vi "Lookup Channel Info.vi"(8 "error in (no error)":errorcluster, 10 "Channel Name":string, 11 "VolatusAPI in":refnum<class "VolatusAPI.lvclass">) -> (0 "error out":errorcluster, 1 "Local":bool, 2 "Channel Info":T1, 3 "VolatusAPI out":refnum<class "VolatusAPI.lvclass">, 4 "Index":i32)   [LabVIEW 2020, in "Volatus.lvlib" / "VolatusAPI.lvclass"]
uses:
  VolatusAPI.lvclass
  lv-vecto/Vecto/Channel Info.ctl
  VolatusAPI.lvclass/VolatusAPI.ctl
  VolatusConfig/VolatusConfig.lvlib
  VolatusConfig/Meta Type.ctl
  lv-cdm/CDM-Config/Config Filter/Config Lookup.lvclass
  VolatusConfig/VolatusConfigElement/VolatusConfigElement.lvclass
  VolatusConfig/Group/Group Config.lvclass
  VolatusConfig/Node/Node Config.lvclass
  C:/dev/lv20CE/relink/lv-volatus/VolatusConfig/VolatusConfigElement/VolatusConfigElement.lvclass
  C:/dev/lv20CE/relink/lv-volatus/VolatusConfig/Node/Node Config.lvclass
  lv-vecto/VectoConfig/VectoConfig.lvlib
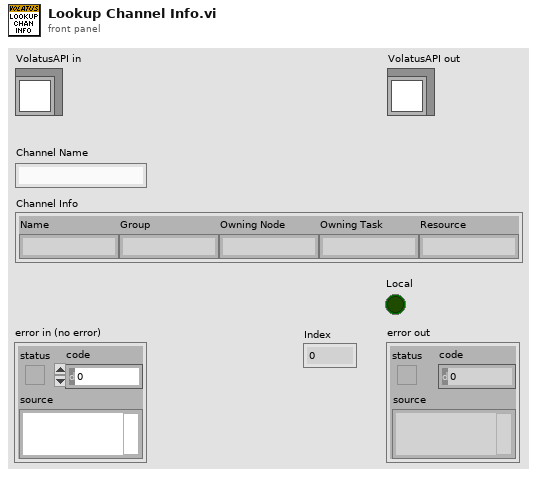
[diagram p1: front panel]
types:
  T1 = typedef "VectoConfig.lvlib/Channel Info.ctl" = cluster{"Name":string, "Group":string, "Owning Node":string, "Owning Task":string, "Resource":string}
  T2 = typedef "VolatusConfig.lvlib/Meta Type.ctl" = enum16{"UNKNOWN", "VL_System", "VL_Cluster", "VL_Node", "VL_Task", "VL_Group", "VL_Channel", "VL_Task_List", "VL_Scaling", "VL_Sensor", "VL_Sensor_List", "VL_Scale"}
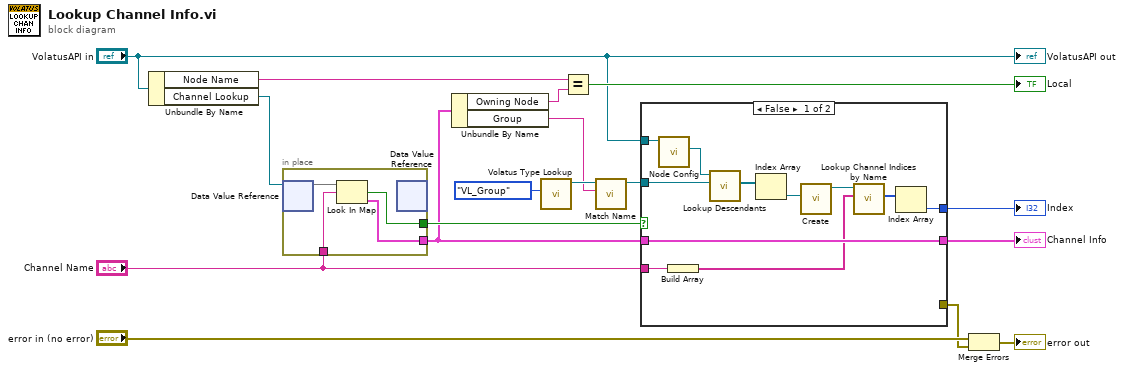
[diagram p0: block diagram]
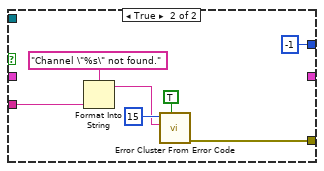
[diagram p2: hidden frame]
diagram:
  n1 = Unbundle By Name("VolatusAPI in") -> ("Node Name"=w9:string, "Channel Lookup"=w14:refnum<data-value>)
  n2 = in-place {
    in-place-border: "Channel Name" -> [w20]
    in-place-border: [w19] -> w10
    in-place-border: [w18] -> w12
    n3 = in-place-dvr #1(w14) -> (w21:map{string, T1})  [unwired: 1 out]
    n4 = Look In Map(map=w21, key=w20) -> (key not found?=w18:bool, value=w19:T1)  [unwired: 1 in]
    n5 = in-place-dvr #1() -> ()  [unwired: 1 in, 2 out]
  }
  n6 = Unbundle By Name(w10) -> ("Owning Node"=w8:string, "Group"=w3:string)
  n7 = call "Volatus Type Lookup.vi"("Meta Type"=Meta_Type."VL_Group") -> ("Config Lookup out"=w4:refnum<class "Config Lookup.lvclass">)  [unwired: 9 in, 1 out]
  n8 = Equal?(x=w9, y=w8) -> (x = y?=→"Local":bool)
  n9 = call "Match Name.vi"("Name"=w3, "Config Lookup (New)"=w4) -> ("Config Lookup out"=w2:refnum<class "Config Lookup.lvclass">)  [unwired: 8 in, 1 out]
  n10 = case shown="False" w12 {
    tunnel: "Channel Name" -> [w25 w35]
    tunnel: [_ w34] -> w15
    tunnel: w10 -> [w32 _]
    tunnel: [w32 _] -> w11
    tunnel: "VolatusAPI in" -> [w31 _]
    tunnel: w2 -> [w30 _]
    tunnel: [w22 -1 ("Numeric")] -> w1
    frame False {
      n11 = call "Node Config.vi"("VolatusAPI in"=w31) -> ("Node Config"=w29:refnum<class "Node Config.lvclass">)  [unwired: 9 in, 1 out]
      n12 = Build Array(w25) -> (w24:string[])
      n13 = call "Lookup Descendants.vi"("Lookup"=w30, "VolatusConfigElement in"=w29) -> ("Descendants"=w28:refnum<class "Config Element.lvclass">[])  [unwired: 7 in, 2 out]
      n14 = Index Array(array=w28) -> (element=w27:refnum<class "Config Element.lvclass">)  [unwired: 1 in]
      n15 = call "Create.vi"("Element"=w27) -> ("Group out"=w26:refnum<class "Group Config.lvclass">)  [unwired: 9 in, 1 out]
      n16 = call "Lookup Channel Indices by Name.vi"("Channel Names"=w24, "Group in"=w26) -> ("Indices"=w23:i32[])  [unwired: 7 in, 2 out]
      n17 = Index Array(array=w23) -> (element=w22:i32)  [unwired: 1 in]
    }
    frame True {
      n18 = Format Into String(format string="Channel \"%s\" not found.", w35) -> (resulting string=w37:string)  [unwired: 2 in, 1 out]
      n19 = call <vilib>:"Error Cluster From Error Code.vi"("show call chain? (False)"=TRUE, "error message (\"\")"=w37, "error code (0)"=15) -> ("error out"=w34:errorcluster)  [unwired: 6 in]
    }
  }
  "Channel Info" <- w11
  "Index" <- w1
  n20 = Merge Errors("error in (no error)", w15) -> (→"error out":errorcluster)
  "VolatusAPI out" <- "VolatusAPI in"
